vi "hw4-4 topVI.vi"() -> ()   [LabVIEW 2014]
panel:
  in  "OFF":bool
  in  "*":bool
  in  ".":bool
  out "INPUT/OUTPUT":string
  in  "b":bool
  in  "c":bool
  in  "/":bool
  in  "-":bool
  in  "+":bool
  in  "0":bool
  in  "9":bool
  in  "6":bool
  in  "8":bool
  in  "5":bool
  in  "7":bool
  in  "4":bool
  in  "3":bool
  in  "2":bool
  in  "1":bool
  in  "=":bool
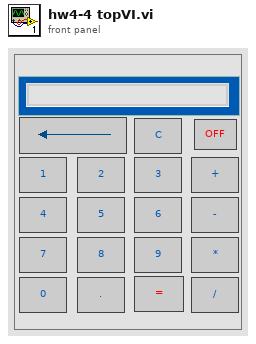
[diagram p1: front panel]
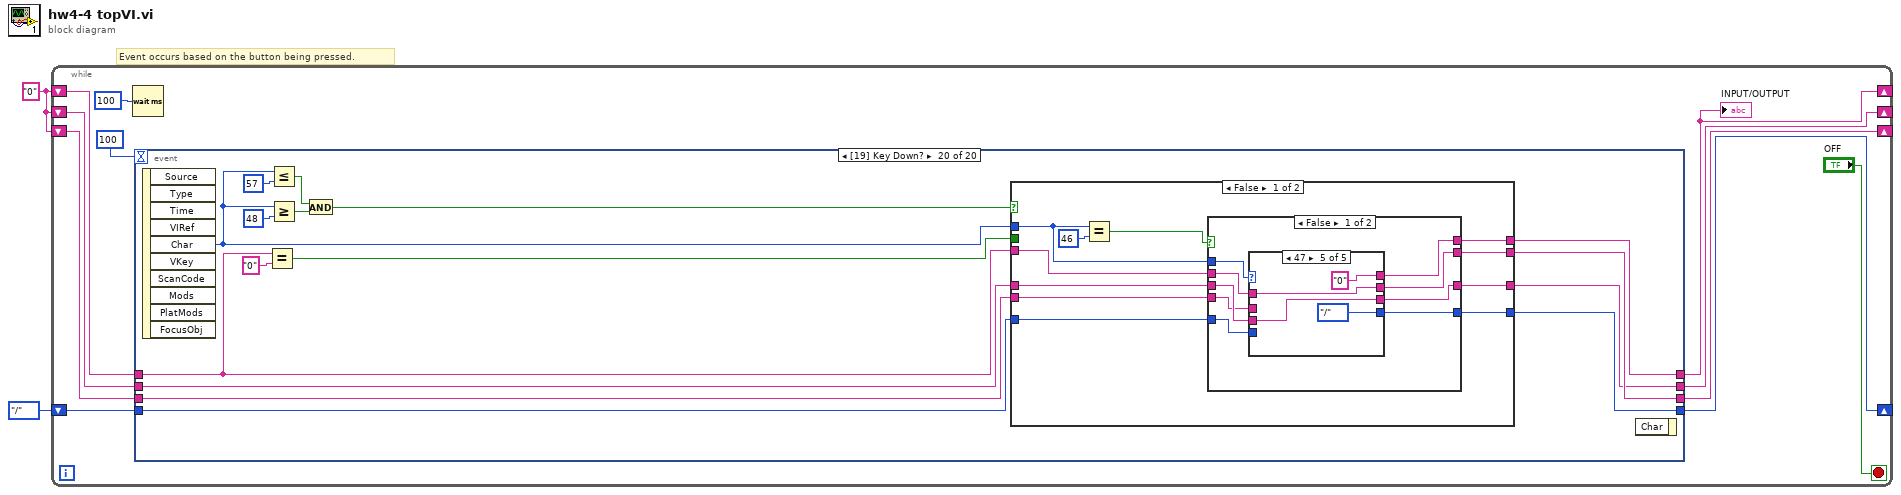
[diagram p0: block diagram]
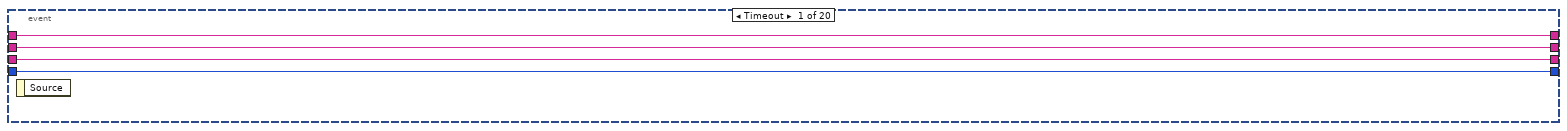
[diagram p2: hidden frame]
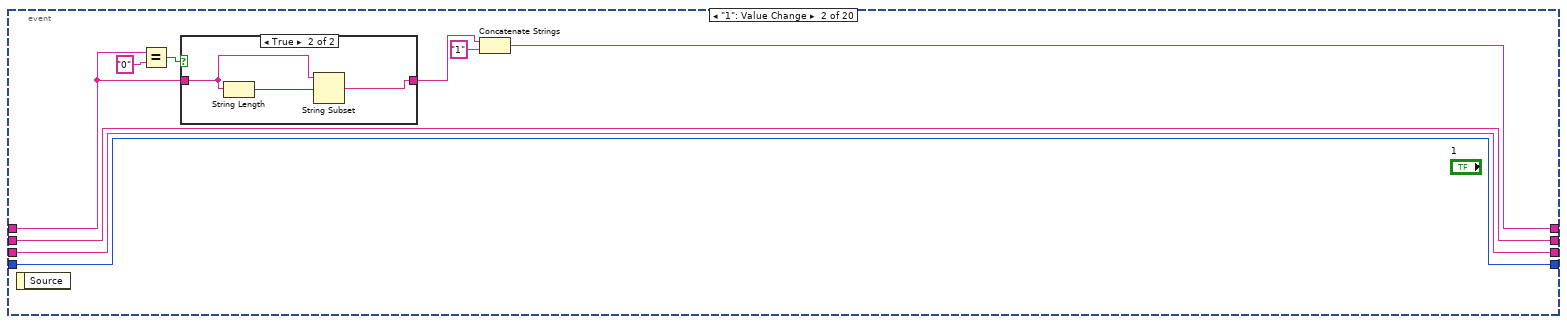
[diagram p3: hidden frame]
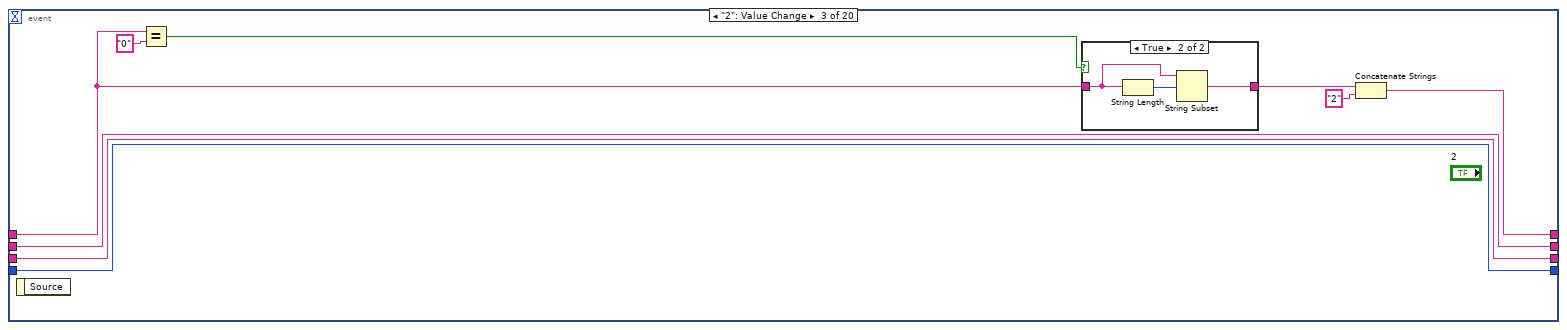
[diagram p5: hidden frame]
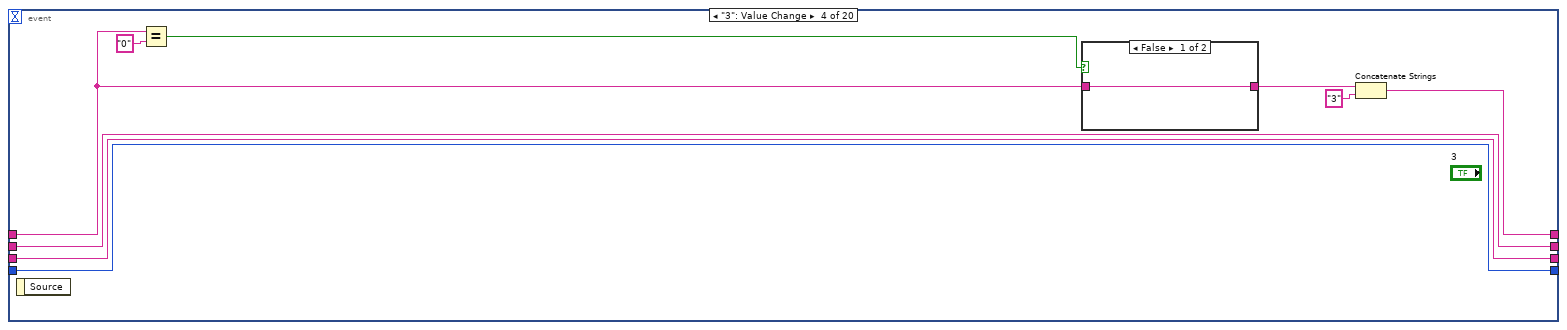
[diagram p7: hidden frame]
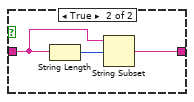
[diagram p8: hidden frame]
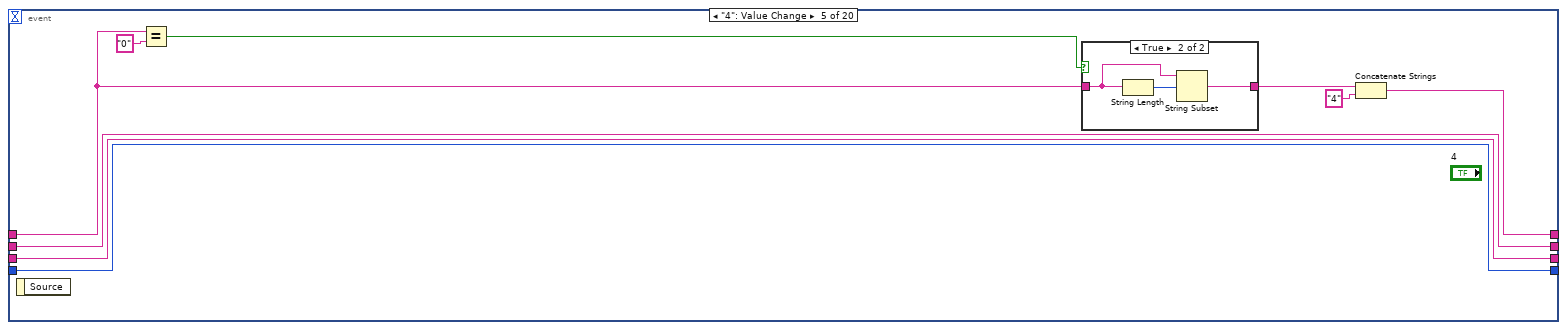
[diagram p9: hidden frame]
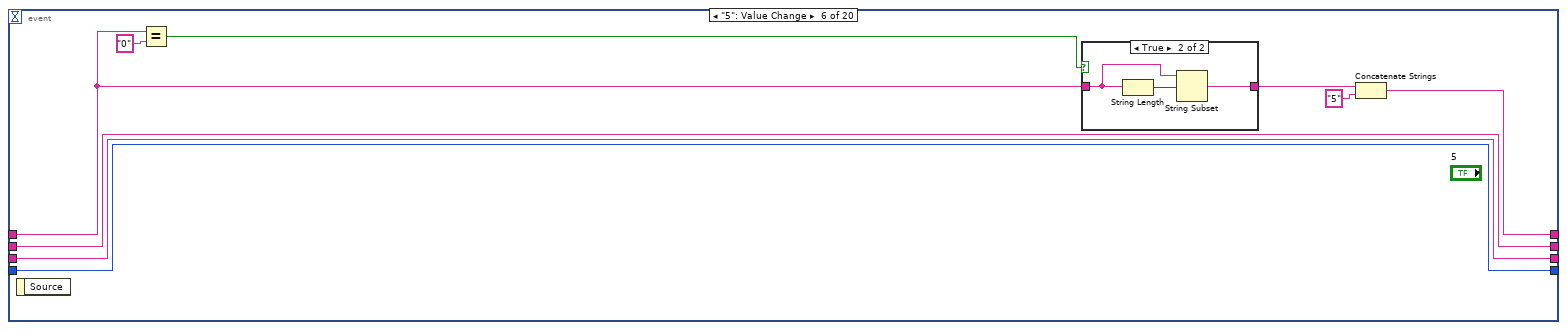
[diagram p11: hidden frame]
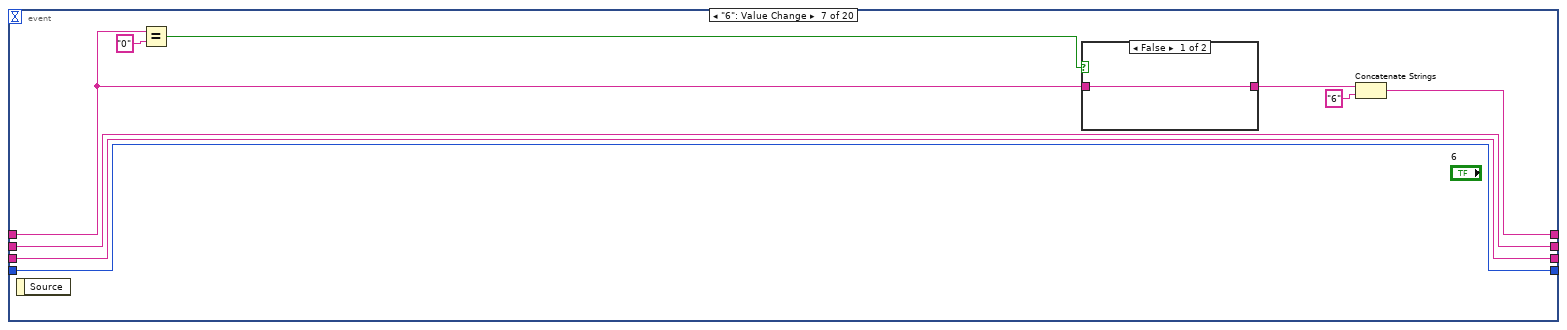
[diagram p13: hidden frame]
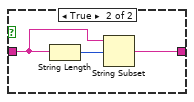
[diagram p14: hidden frame]
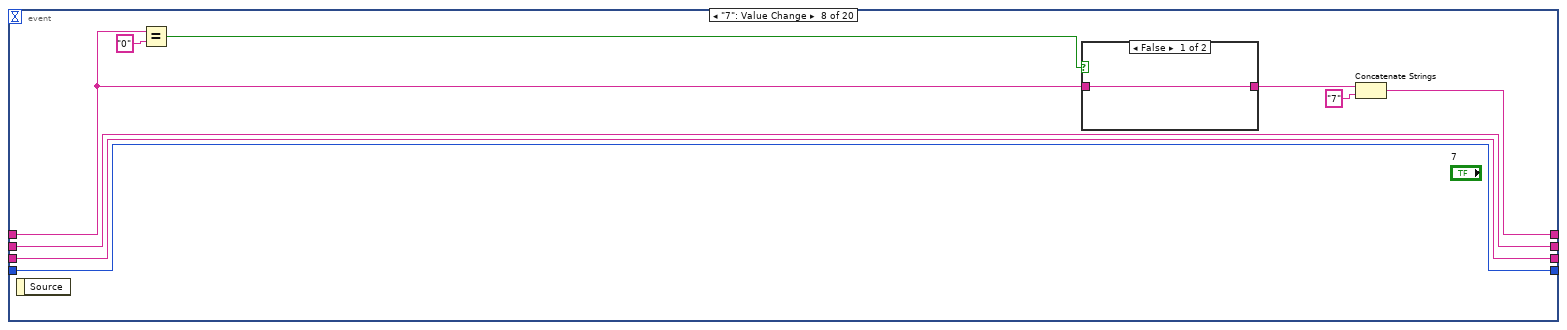
[diagram p15: hidden frame]
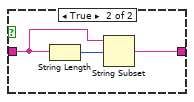
[diagram p16: hidden frame]
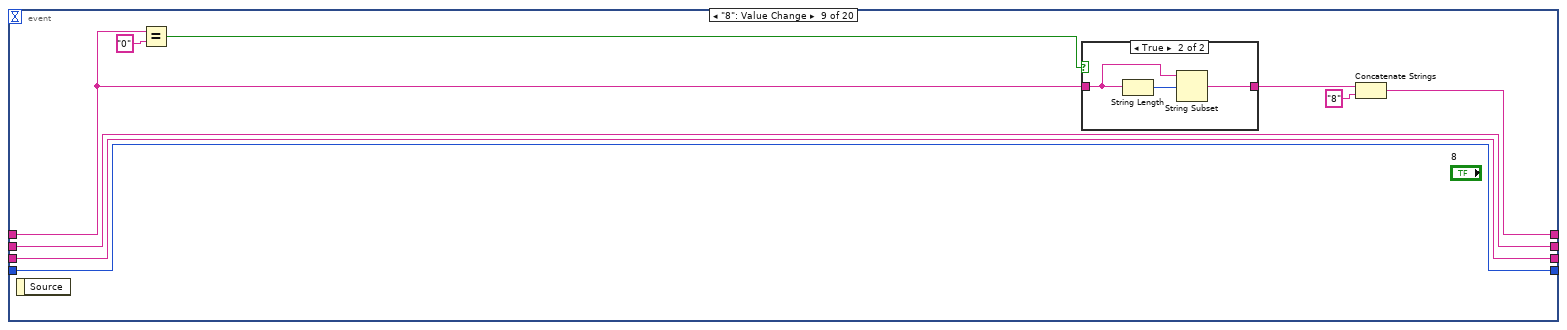
[diagram p17: hidden frame]
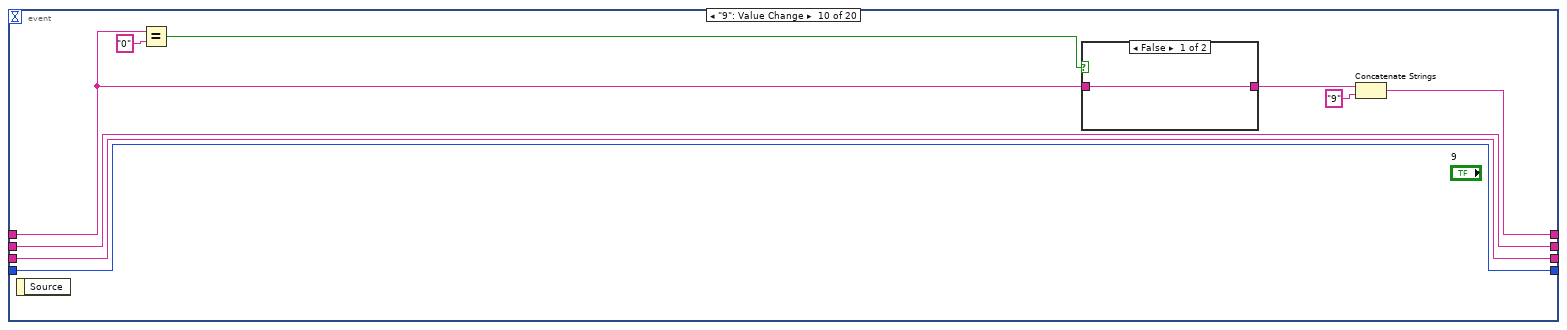
[diagram p19: hidden frame]
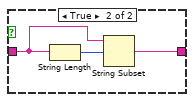
[diagram p20: hidden frame]
diagram:
  w1 = "0"
  # "Event occurs based on the button being pressed."
  n1 = while {
    shift-right: [w6] -> _
    shift-left: w1 -> [w13]
    shift-right: [w12] -> _
    shift-left: w1 -> [w11]
    shift-right: [w8] -> _
    shift-left: enum16{"+", "-", "*", "/"}."/" -> [w7]
    shift-right: [w5] -> _
    shift-left: w1 -> [w4]
    stop <- "OFF" stop-if-true
    n2 = Wait (ms)(milliseconds to wait=u32 100 ("millisecond multiple")) -> ()  [unwired: 1 out]
    n3 = event shown="[19] Key Down?" {
      selector: _ -> [_ _ _ _ _ _ _ _ _ _ _ _ _ _ _ _ _ _ _ _]
      dyn-events: _ -> [_ _ _ _ _ _ _ _ _ _ _ _ _ _ _ _ _ _ _ _]
      timeout: 100 -> [_ _ _ _ _ _ _ _ _ _ _ _ _ _ _ _ _ _ _ _]
      tunnel: w13 -> [w15 w19 w32 w45 w59 w71 w84 w97 w110 w123 w140 w141 w153 w157 w160 w164 w168 w177 w236 w252]
      tunnel: [w17 w25 w38 w51 w64 w77 w91 w103 w116 w129 w138 w143 w148 w157 w160 w164 w168 "0" w238 w240] -> w12
      tunnel: w11 -> [w17 w25 w38 w51 w64 w77 w91 w103 w116 w129 w138 w143 w148 _ _ _ _ w170 w238 w241]
      tunnel: w7 -> [w16 w24 w37 w50 w63 w76 w90 w102 w115 w128 w137 w144 w147 _ _ _ _ w179 w237 w251]
      tunnel: [w16 w24 w37 w50 w63 w76 w90 w102 w115 w128 w137 w144 w147 enum16{"+", "-", "*", "/"}."+" enum16{"+", "-", "*", "/"}."-" enum16{"+", "-", "*", "/"}."*" enum16{"+", "-", "*", "/"}."/" w178 w237 w250] -> w8
      tunnel: [w15 w23 w36 w49 w62 w75 w89 w101 w114 w127 w136 "0" w146 "0" "0" "0" "0" w173 w235 w243] -> w6
      tunnel: [w14 w18 w31 w44 w57 w70 w83 w96 w109 w122 w135 w141 w145 w154 w158 w162 w166 w172 w233 w239] -> w5
      tunnel: w4 -> [w14 w18 w31 w44 w57 w70 w83 w96 w109 w122 w135 _ w145 w154 w158 w162 w166 w172 w233 w242]
      event Timeout {
        n4 = event-data() -> ()  [unwired: 1 in, 1 out]
      }
      event "1": Value Change {
        n5 = event-data() -> ()  [unwired: 1 in, 1 out]
        n6 = Equal?(x=w19, y="0") -> (x = y?=w22:bool)
        n7 = case shown="True" w22 {
          tunnel: w19 -> [w27 w29]
          tunnel: [w27 w28] -> w20
          frame False {
          }
          frame True {
            n8 = String Length(string=w29) -> (length=w30:i32)
            n9 = String Subset(string=w29, offset (0)=w30) -> (substring=w28:string)  [unwired: 1 in]
          }
        }
        n10 = Concatenate Strings "Concatenate Strings"(w20, "1") -> (w23:string)
      }
      event "2": Value Change {
        n11 = event-data() -> ()  [unwired: 1 in, 1 out]
        n12 = Equal?(x=w32, y="0") -> (x = y?=w35:bool)
        n13 = case shown="True" w35 {
          tunnel: w32 -> [w40 w42]
          tunnel: [w40 w41] -> w33
          frame False {
          }
          frame True {
            n14 = String Length(string=w42) -> (length=w43:i32)
            n15 = String Subset(string=w42, offset (0)=w43) -> (substring=w41:string)  [unwired: 1 in]
          }
        }
        n16 = Concatenate Strings(w33, "2") -> (w36:string)
      }
      event "3": Value Change {
        n17 = event-data() -> ()  [unwired: 1 in, 1 out]
        n18 = Equal?(x=w45, y="0") -> (x = y?=w48:bool)
        n19 = case shown="False" w48 {
          tunnel: w45 -> [w53 w55]
          tunnel: [w53 w54] -> w46
          frame False {
          }
          frame True {
            n20 = String Length(string=w55) -> (length=w56:i32)
            n21 = String Subset(string=w55, offset (0)=w56) -> (substring=w54:string)  [unwired: 1 in]
          }
        }
        n22 = Concatenate Strings(w46, "3") -> (w49:string)
      }
      event "4": Value Change {
        n23 = event-data() -> ()  [unwired: 1 in, 1 out]
        n24 = Equal?(x=w59, y="0") -> (x = y?=w61:bool)
        n25 = case shown="True" w61 {
          tunnel: w59 -> [w66 w68]
          tunnel: [w66 w67] -> w58
          frame False {
          }
          frame True {
            n26 = String Length(string=w68) -> (length=w69:i32)
            n27 = String Subset(string=w68, offset (0)=w69) -> (substring=w67:string)  [unwired: 1 in]
          }
        }
        n28 = Concatenate Strings(w58, "4") -> (w62:string)
      }
      event "5": Value Change {
        n29 = event-data() -> ()  [unwired: 1 in, 1 out]
        n30 = Equal?(x=w71, y="0") -> (x = y?=w74:bool)
        n31 = case shown="True" w74 {
          tunnel: w71 -> [w79 w81]
          tunnel: [w79 w80] -> w72
          frame False {
          }
          frame True {
            n32 = String Length(string=w81) -> (length=w82:i32)
            n33 = String Subset(string=w81, offset (0)=w82) -> (substring=w80:string)  [unwired: 1 in]
          }
        }
        n34 = Concatenate Strings(w72, "5") -> (w75:string)
      }
      event "6": Value Change {
        n35 = event-data() -> ()  [unwired: 1 in, 1 out]
        n36 = Equal?(x=w84, y="0") -> (x = y?=w87:bool)
        n37 = case shown="False" w87 {
          tunnel: w84 -> [w92 w94]
          tunnel: [w92 w93] -> w85
          frame False {
          }
          frame True {
            n38 = String Length(string=w94) -> (length=w95:i32)
            n39 = String Subset(string=w94, offset (0)=w95) -> (substring=w93:string)  [unwired: 1 in]
          }
        }
        n40 = Concatenate Strings(w85, "6") -> (w89:string)
      }
      event "7": Value Change {
        n41 = event-data() -> ()  [unwired: 1 in, 1 out]
        n42 = Equal?(x=w97, y="0") -> (x = y?=w100:bool)
        n43 = case shown="False" w100 {
          tunnel: w97 -> [w105 w107]
          tunnel: [w105 w106] -> w98
          frame False {
          }
          frame True {
            n44 = String Length(string=w107) -> (length=w108:i32)
            n45 = String Subset(string=w107, offset (0)=w108) -> (substring=w106:string)  [unwired: 1 in]
          }
        }
        n46 = Concatenate Strings(w98, "7") -> (w101:string)
      }
      event "8": Value Change {
        n47 = event-data() -> ()  [unwired: 1 in, 1 out]
        n48 = Equal?(x=w110, y="0") -> (x = y?=w113:bool)
        n49 = case shown="True" w113 {
          tunnel: w110 -> [w118 w120]
          tunnel: [w118 w119] -> w111
          frame False {
          }
          frame True {
            n50 = String Length(string=w120) -> (length=w121:i32)
            n51 = String Subset(string=w120, offset (0)=w121) -> (substring=w119:string)  [unwired: 1 in]
          }
        }
        n52 = Concatenate Strings(w111, "8") -> (w114:string)
      }
      event "9": Value Change {
        n53 = event-data() -> ()  [unwired: 1 in, 1 out]
        n54 = Equal?(x=w123, y="0") -> (x = y?=w126:bool)
        n55 = case shown="False" w126 {
          tunnel: w123 -> [w131 w133]
          tunnel: [w131 w132] -> w124
          frame False {
          }
          frame True {
            n56 = String Length(string=w133) -> (length=w134:i32)
            n57 = String Subset(string=w133, offset (0)=w134) -> (substring=w132:string)  [unwired: 1 in]
          }
        }
        n58 = Concatenate Strings(w124, "9") -> (w127:string)
      }
      event "0": Value Change {
        n59 = event-data() -> ()  [unwired: 1 in, 1 out]
        n60 = Concatenate Strings(w140, "0") -> (w136:string)
      }
      event "c": Value Change {
        n61 = event-data() -> ()  [unwired: 1 in, 1 out]
      }
      event "b": Value Change {
        n62 = event-data() -> ()  [unwired: 1 in, 1 out]
        n63 = Reverse String(1:w153) -> (0:w149:string)
        n64 = String Length(string=w149) -> (length=w150:i32)
        n65 = String Subset(string=w149, offset (0)=1, length (rest)=w150) -> (substring=w151:string)
        n66 = Reverse String(1:w151) -> (0:w146:string)
      }
      event "+": Value Change {
        n67 = event-data() -> ()  [unwired: 1 in, 1 out]
      }
      event "-": Value Change {
        n68 = event-data() -> ()  [unwired: 1 in, 1 out]
      }
      event "*": Value Change {
        n69 = event-data() -> ()  [unwired: 1 in, 1 out]
      }
      event "/": Value Change {
        n70 = event-data() -> ()  [unwired: 1 in, 1 out]
      }
      event "=": Value Change {
        n71 = event-data() -> ()  [unwired: 1 in, 1 out]
        n72 = case shown="\"+\"" w179 {
          selector: w179 -> [w211 w218 w225 w232]
          tunnel: [w211 w218 w225 w232] -> w178
          tunnel: w170 -> [w207 w215 w220 w227]
          tunnel: w177 -> [w206 w216 w221 w228]
          tunnel: [w205 w214 w219 w226] -> w174
          frame "+" {
            n73 = Fract/Exp String To Number(string=w206) -> (number=w209:dbl)  [unwired: 3 in, 1 out]
            n74 = Fract/Exp String To Number(string=w207) -> (number=w210:dbl)  [unwired: 3 in, 1 out]
            n75 = Add(x=w210, y=w209) -> (x+y=w208:dbl)
            n76 = Number To Fractional String(number=w208) -> (F-format string=w205:string)  [unwired: 3 in]
          }
          frame "-" {
            n77 = Fract/Exp String To Number(string=w216) -> (number=w212:dbl)  [unwired: 3 in, 1 out]
            n78 = Fract/Exp String To Number(string=w215) -> (number=w213:dbl)  [unwired: 3 in, 1 out]
            n79 = Subtract(x=w213, y=w212) -> (x-y=w217:dbl)
            n80 = Number To Fractional String(number=w217) -> (F-format string=w214:string)  [unwired: 3 in]
          }
          frame "*" {
            n81 = Fract/Exp String To Number(string=w221) -> (number=w223:dbl)  [unwired: 3 in, 1 out]
            n82 = Fract/Exp String To Number(string=w220) -> (number=w224:dbl)  [unwired: 3 in, 1 out]
            n83 = Multiply(x=w224, y=w223) -> (x*y=w222:dbl)
            n84 = Number To Fractional String(number=w222) -> (F-format string=w219:string)  [unwired: 3 in]
          }
          frame "/" {
            n85 = Fract/Exp String To Number(string=w228) -> (number=w230:dbl)  [unwired: 3 in, 1 out]
            n86 = Fract/Exp String To Number(string=w227) -> (number=w231:dbl)  [unwired: 3 in, 1 out]
            n87 = Divide(x=w231, y=w230) -> (x/y=w229:dbl)
            n88 = Number To Fractional String(number=w229) -> (F-format string=w226:string)  [unwired: 3 in]
          }
        }
        n89 = String Length(string=w174) -> (length=w176:i32)
        n90 = for {
          N: w176 -> [_]
          tunnel: w174 -> [w189]
          shift-right: [w188] -> _
          shift-left: "" -> [w192]
          tunnel: [w181] -> w173
          i -> [w194]
          stop <- w183 stop-if-true
          n91 = Reverse String(1:w189) -> (0:w190:string)
          n92 = String Subset(string=w190, offset (0)=w194, length (rest)=1 ("length (rest)")) -> (substring=w186:string)
          n93 = Equal?(x=w186, y=".") -> (x = y?=w180:bool)
          n94 = Greater?(x=w186, y="0") -> (0:w184:bool)
          n95 = Or(x=w180, y=w184) -> (x .or. y?=w183:bool)
          n96 = case shown="False" w183 {
            tunnel: w192 -> [w203 w204]
            tunnel: w186 -> [w202 _]
            tunnel: [w201 w204] -> w188
            frame False {
              n97 = Concatenate Strings(w203, w202) -> (w201:string)
            }
            frame True {
            }
          }
          n98 = Reverse String(1:w188) -> (0:w187:string)
          n99 = Match Pattern(string=w189, regular expression=w187) -> (before substring=w182:string)  [unwired: 1 in, 3 out]
          n100 = case shown="False" w180 {
            tunnel: w182 -> [w195 w200]
            tunnel: [w195 w196] -> w181
            frame False {
            }
            frame True {
              n101 = Reverse String(1:w200) -> (0:w198:string)
              n102 = Match Pattern(string=w198, regular expression=".") -> (after substring=w197:string)  [unwired: 1 in, 3 out]
              n103 = Reverse String(1:w197) -> (0:w196:string)
            }
          }
        }
      }
      event ".": Value Change {
        n104 = event-data() -> ()  [unwired: 1 in, 1 out]
        n105 = Concatenate Strings(w236, "." ("string")) -> (w235:string)
      }
      event Key Down? {
        n106 = event-data() -> ("Char"=w247:i16)  [unwired: 1 in, 9 out]
        n107 = Equal?(x=w252, y="0") -> (x = y?=w253:bool)
        n108 = Less Or Equal?(x=w247, y=57) -> (x <= y?=w246:bool)
        n109 = Greater Or Equal?(x=w247, y=48) -> (x >= y?=w245:bool)
        n110 = And(x=w246, y=w245) -> (x .and. y?=w244:bool)
        n111 = case shown="False" w244 {
          tunnel: w253 -> [_ w308]
          tunnel: w252 -> [w261 w307]
          tunnel: [w259 w305] -> w243
          tunnel: w247 -> [w260 w304]
          tunnel: w251 -> [w263 w303]
          tunnel: [w262 w303] -> w250
          tunnel: w242 -> [w258 w302]
          tunnel: w241 -> [w257 w301]
          tunnel: [w256 w301] -> w240
          tunnel: [w255 w302] -> w239
          frame False {
            n112 = Equal?(x=w260, y=i16 46) -> (x = y?=w264:bool)
            n113 = case shown="False" w264 {
              tunnel: w263 -> [w271 w300]
              tunnel: [w273 w300] -> w262
              tunnel: w261 -> [w272 w299]
              tunnel: [w270 w298] -> w259
              tunnel: w260 -> [w274 _]
              tunnel: w258 -> [w267 w296]
              tunnel: w257 -> [w266 w295]
              tunnel: [w268 w295] -> w256
              tunnel: [w269 w296] -> w255
              frame False {
                n114 = case shown="47" w274 {
                  tunnel: [w277 enum16{"+", "-", "*", "/"}."*" enum16{"+", "-", "*", "/"}."+" enum16{"+", "-", "*", "/"}."-" enum16{"+", "-", "*", "/"}."/"] -> w273
                  tunnel: [w278 "0" "0" "0" "0"] -> w270
                  tunnel: w272 -> [w278 w280 w283 w288 w292]
                  tunnel: w271 -> [w277 _ _ _ _]
                  tunnel: [w275 w279 w284 w287 w291] -> w269
                  tunnel: w266 -> [w276 _ _ _ _]
                  tunnel: [w276 w280 w283 w288 w292] -> w268
                  tunnel: w267 -> [w275 w279 w284 w287 w291]
                  frame Default {
                  }
                  frame 42 {
                  }
                  frame 43 {
                  }
                  frame 45 {
                  }
                  frame 47 {
                  }
                }
              }
              frame True {
                n115 = Concatenate Strings(w299, "." ("string")) -> (w298:string)
              }
            }
          }
          frame True {
            n116 = case shown="True" w308 {
              tunnel: w307 -> [w309 w311]
              tunnel: [w309 w310] -> w306
              frame False {
              }
              frame True {
                n117 = String Length(string=w311) -> (length=w312:i32)
                n118 = String Subset(string=w311, offset (0)=w312) -> (substring=w310:string)  [unwired: 1 in]
              }
            }
            n119 = case shown="51" w304 {
              tunnel: w306 -> [w313 w316 w319 w322 w325 w328 w331 w334 w337 w340 w343]
              tunnel: [w313 w314 w317 w320 w323 w326 w329 w332 w335 w338 w341] -> w305
              frame Default {
              }
              frame 49 {
                n120 = Concatenate Strings(w316, "1") -> (w314:string)
              }
              frame 50 {
                n121 = Concatenate Strings(w319, "2") -> (w317:string)
              }
              frame 51 {
                n122 = Concatenate Strings(w322, "3") -> (w320:string)
              }
              frame 52 {
                n123 = Concatenate Strings(w325, "4") -> (w323:string)
              }
              frame 53 {
                n124 = Concatenate Strings(w328, "5") -> (w326:string)
              }
              frame 54 {
                n125 = Concatenate Strings(w331, "6") -> (w329:string)
              }
              frame 55 {
                n126 = Concatenate Strings(w334, "7") -> (w332:string)
              }
              frame 56 {
                n127 = Concatenate Strings(w337, "8") -> (w335:string)
              }
              frame 57 {
                n128 = Concatenate Strings(w340, "9") -> (w338:string)
              }
              frame 48 {
                n129 = Concatenate Strings(w343, "0") -> (w341:string)
              }
            }
          }
        }
        n130 = event-data() -> ()  [unwired: 2 in, 1 out]
      }
    }
    "INPUT/OUTPUT" <- w6
  }
